vi "dfd_FIR Windowed (Uniform) Filter Coefficients.vi"(6 "sampling freq: fs":dbl=1.0 format="%0.2f", 7 "filter type":T1(ring), 8 "error in (no error)":errorcluster, 9 "low cutoff freq: fl":dbl=0.125 format="%0.2f", 10 "high cutoff freq: fh":dbl=0.45 format="%0.2f", 11 "order":i32=25) -> (0 "error out":errorcluster, 3 "FIR Coefficients":dbl[](array[numeric]) format="%#_2f")   [LabVIEW 2017, in "NI_DigFilter_Design.lvlib"]
doc: "Generates the set of coefficients to implement an FIR filter."
uses:
  <vilib>/addons/Digital Filter Design/NI_DigFilter_Design.lvlib
  <vilib>/Analysis/1siggen.llb/Ramp Pattern by Samples.vi
  <vilib>/Analysis/NI_AALBase.lvlib
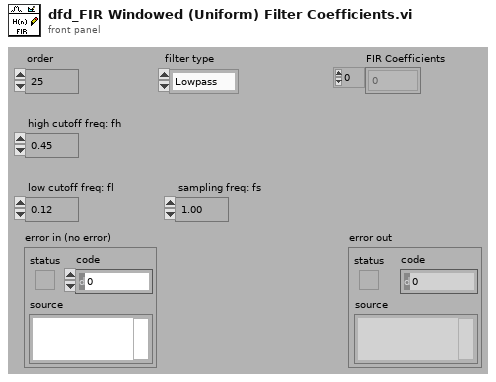
[diagram p1: front panel]
types:
  T1 = enum16{"Lowpass", "Highpass", "Bandpass", "Bandstop"}
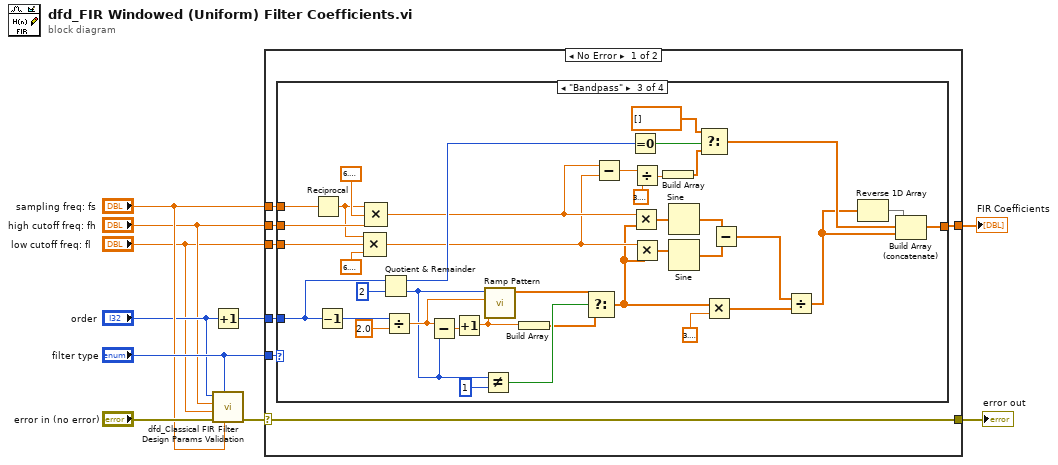
[diagram p0: block diagram]
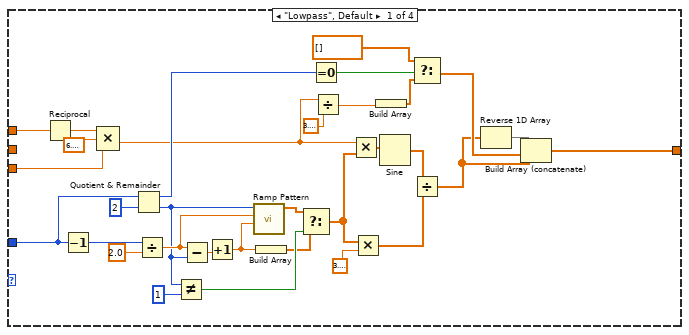
[diagram p2: hidden frame]
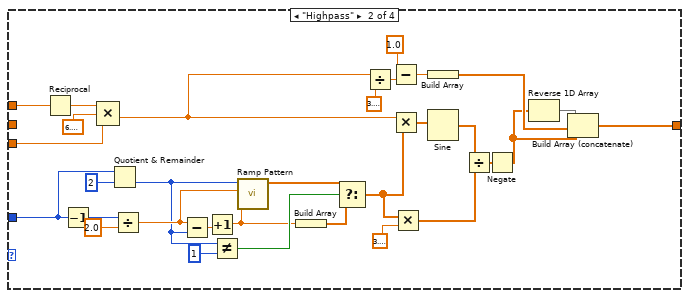
[diagram p3: hidden frame]
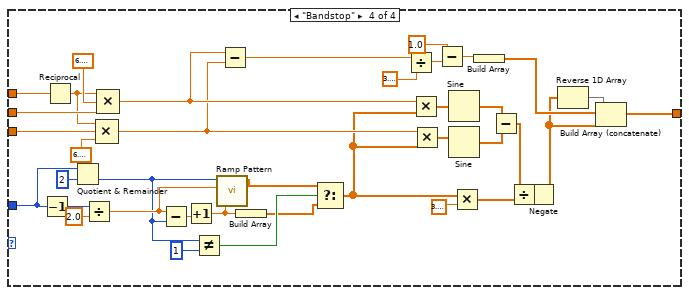
[diagram p4: hidden frame]
diagram:
  n1 = Increment(x="order") -> (x+1=w1:i32)
  n2 = call <vilib>:"dfd_Classical FIR Filter Design Params Validation.vi"("fs [Hz]"="sampling freq: fs", "filter type"="filter type", "error in (no error)"="error in (no error)", "low cutoff freq: fl"="low cutoff freq: fl", "high cutoff freq: fh"="high cutoff freq: fh", "order"="order") -> ("error out"=w3:errorcluster)  [unwired: 5 out]
  n3 = case shown="No Error" w3 {
    selector: w3 -> [w11 w158]
    tunnel: [w17 _] -> w10
    tunnel: "filter type" -> [w16 _]
    tunnel: "sampling freq: fs" -> [w15 _]
    tunnel: w1 -> [w14 _]
    tunnel: "high cutoff freq: fh" -> [w13 _]
    tunnel: "low cutoff freq: fl" -> [w12 _]
    tunnel: [w11 w158] -> w2
    frame No Error {
      n4 = case shown="\"Bandpass\"" w16 {
        tunnel: w15 -> [w49 w80 w117 w155]
        tunnel: w13 -> [_ _ w118 w156]
        tunnel: w14 -> [w45 w76 w82 w145]
        tunnel: [w29 w65 w92 w134] -> w17
        tunnel: w12 -> [w25 w57 w114 w152]
        frame "Lowpass", Default {
          n5 = Reciprocal(x=w49) -> (1/x=w48:dbl)
          n6 = Decrement(x=w45) -> (x-1=w27:i32)
          n7 = Compound Arithmetic op=MULTIPLY(w48, 6.283185307179586, w25) -> (w33:dbl)
          n8 = Quotient & Remainder(x=w45, y=2) -> (x-y*floor(x/y)=w37:i32, floor(x/y)=w24:i32)
          n9 = Divide(x=w27, y=2.0) -> (x/y=w43:dbl)
          n10 = Not Equal?(x=w24, y=1) -> (x != y?=w22:bool)
          n11 = Subtract(x=w43, y=w24) -> (x-y=w42:dbl)
          n12 = Increment(x=w42) -> (x+1=w19:dbl)
          n13 = call-poly <vilib>:"Ramp Pattern.vi"("start"=w19, "end"=w43, "samples"=w24) -> ("Ramp Pattern"=w21:dbl[])  [unwired: 7 in, 1 out]
          n14 = Build Array(w19) -> (w18:dbl[])
          n15 = Select(t=w21, s=w22, f=w18) -> (s? t:f=w20:dbl[])
          n16 = Equal To 0?(x=w37) -> (x = 0?=w36:bool)
          n17 = Divide(x=w33, y=3.141592653589793) -> (x/y=w32:dbl)
          n18 = Multiply(x=w33, y=w20) -> (x*y=w40:dbl[])
          n19 = Multiply(x=w20, y=3.141592653589793) -> (x*y=w38:dbl[])
          n20 = Build Array(w32) -> (w31:dbl[])
          n21 = Sine(x=w40) -> (sin(x)=w39:dbl[])
          n22 = Select(t=dbl[] [], s=w36, f=w31) -> (s? t:f=w30:dbl[])
          n23 = Divide(x=w39, y=w38) -> (x/y=w26:dbl[])
          n24 = Reverse 1D Array(array=w26) -> (reversed array=w28:dbl[])
          n25 = Build Array (concatenate)(w28, w30, w26) -> (w29:dbl[])
        }
        frame "Highpass" {
          n26 = Reciprocal(x=w80) -> (1/x=w79:dbl)
          n27 = Decrement(x=w76) -> (x-1=w62:i32)
          n28 = Compound Arithmetic op=MULTIPLY(w79, 6.283185307179586, w57) -> (w67:dbl)
          n29 = Quotient & Remainder(x=w76, y=2) -> (floor(x/y)=w55:i32)  [unwired: 1 out]
          n30 = Divide(x=w62, y=2.0) -> (x/y=w74:dbl)
          n31 = Subtract(x=w74, y=w55) -> (x-y=w73:dbl)
          n32 = Increment(x=w73) -> (x+1=w51:dbl)
          n33 = Not Equal?(x=w55, y=1) -> (x != y?=w52:bool)
          n34 = call-poly <vilib>:"Ramp Pattern.vi"("start"=w51, "end"=w74, "samples"=w55) -> ("Ramp Pattern"=w53:dbl[])  [unwired: 7 in, 1 out]
          n35 = Build Array(w51) -> (w50:dbl[])
          n36 = Select(t=w53, s=w52, f=w50) -> (s? t:f=w54:dbl[])
          n37 = Divide(x=w67, y=3.141592653589793) -> (x/y=w66:dbl)
          n38 = Subtract(x=1.0 ("y"), y=w66) -> (x-y=w61:dbl)
          n39 = Multiply(x=w67, y=w54) -> (x*y=w71:dbl[])
          n40 = Multiply(x=w54, y=3.141592653589793) -> (x*y=w69:dbl[])
          n41 = Build Array(w61) -> (w59:dbl[])
          n42 = Sine(x=w71) -> (sin(x)=w70:dbl[])
          n43 = Divide(x=w70, y=w69) -> (x/y=w64:dbl[])
          n44 = Negate(x=w64) -> (-x=w58:dbl[])
          n45 = Reverse 1D Array(array=w58) -> (reversed array=w63:dbl[])
          n46 = Build Array (concatenate)(w63, w59, w58) -> (w65:dbl[])
        }
        frame "Bandpass" {
          n47 = Reciprocal(x=w117) -> (1/x=w116:dbl)
          n48 = Decrement(x=w82) -> (x-1=w81:i32)
          n49 = Compound Arithmetic op=MULTIPLY(w116, w114, 6.283185307179586) -> (w90:dbl)
          n50 = Compound Arithmetic op=MULTIPLY(w116, 6.283185307179586, w118) -> (w91:dbl)
          n51 = Quotient & Remainder(x=w82, y=2) -> (x-y*floor(x/y)=w97:i32, floor(x/y)=w88:i32)
          n52 = Divide(x=w81, y=2.0) -> (x/y=w111:dbl)
          n53 = Subtract(x=w111, y=w88) -> (x-y=w112:dbl)
          n54 = Increment(x=w112) -> (x+1=w84:dbl)
          n55 = Not Equal?(x=w88, y=1) -> (x != y?=w85:bool)
          n56 = call-poly <vilib>:"Ramp Pattern.vi"("start"=w84, "end"=w111, "samples"=w88) -> ("Ramp Pattern"=w86:dbl[])  [unwired: 7 in, 1 out]
          n57 = Build Array(w84) -> (w83:dbl[])
          n58 = Select(t=w86, s=w85, f=w83) -> (s? t:f=w87:dbl[])
          n59 = Subtract(x=w91, y=w90) -> (x-y=w96:dbl)
          n60 = Equal To 0?(x=w97) -> (x = 0?=w98:bool)
          n61 = Multiply(x=w91, y=w87) -> (x*y=w108:dbl[])
          n62 = Divide(x=w96, y=3.141592653589793) -> (x/y=w101:dbl)
          n63 = Multiply(x=w90, y=w87) -> (x*y=w107:dbl[])
          n64 = Build Array(w101) -> (w102:dbl[])
          n65 = Sine(x=w108) -> (sin(x)=w106:dbl[])
          n66 = Sine(x=w107) -> (sin(x)=w105:dbl[])
          n67 = Select(t=dbl[] [], s=w98, f=w102) -> (s? t:f=w94:dbl[])
          n68 = Multiply(x=w87, y=3.141592653589793) -> (x*y=w103:dbl[])
          n69 = Subtract(x=w106, y=w105) -> (x-y=w104:dbl[])
          n70 = Divide(x=w104, y=w103) -> (x/y=w93:dbl[])
          n71 = Reverse 1D Array(array=w93) -> (reversed array=w95:dbl[])
          n72 = Build Array (concatenate)(w95, w94, w93) -> (w92:dbl[])
        }
        frame "Bandstop" {
          n73 = Decrement(x=w145) -> (x-1=w151:i32)
          n74 = Reciprocal(x=w155) -> (1/x=w154:dbl)
          n75 = Quotient & Remainder(x=w145, y=2) -> (floor(x/y)=w127:i32)  [unwired: 1 out]
          n76 = Divide(x=w151, y=2.0) -> (x/y=w148:dbl)
          n77 = Compound Arithmetic op=MULTIPLY(w154, w152, 6.283185307179586) -> (w132:dbl)
          n78 = Compound Arithmetic op=MULTIPLY(w154, 6.283185307179586, w156) -> (w133:dbl)
          n79 = Subtract(x=w148, y=w127) -> (x-y=w149:dbl)
          n80 = Increment(x=w149) -> (x+1=w123:dbl)
          n81 = Not Equal?(x=w127, y=1) -> (x != y?=w124:bool)
          n82 = call-poly <vilib>:"Ramp Pattern.vi"("start"=w123, "end"=w148, "samples"=w127) -> ("Ramp Pattern"=w126:dbl[])  [unwired: 7 in, 1 out]
          n83 = Subtract(x=w133, y=w132) -> (x-y=w137:dbl)
          n84 = Build Array(w123) -> (w122:dbl[])
          n85 = Select(t=w126, s=w124, f=w122) -> (s? t:f=w125:dbl[])
          n86 = Divide(x=w137, y=3.141592653589793) -> (x/y=w139:dbl)
          n87 = Multiply(x=w133, y=w125) -> (x*y=w144:dbl[])
          n88 = Multiply(x=w132, y=w125) -> (x*y=w143:dbl[])
          n89 = Subtract(x=1.0, y=w139) -> (x-y=w130:dbl)
          n90 = Sine(x=w144) -> (sin(x)=w142:dbl[])
          n91 = Sine(x=w143) -> (sin(x)=w141:dbl[])
          n92 = Multiply(x=w125, y=3.141592653589793) -> (x*y=w140:dbl[])
          n93 = Build Array(w130) -> (w131:dbl[])
          n94 = Subtract(x=w142, y=w141) -> (x-y=w121:dbl[])
          n95 = Divide(x=w121, y=w140) -> (x/y=w135:dbl[])
          n96 = Negate(x=w135) -> (-x=w120:dbl[])
          n97 = Reverse 1D Array(array=w120) -> (reversed array=w136:dbl[])
          n98 = Build Array (concatenate)(w136, w131, w120) -> (w134:dbl[])
        }
      }
    }
    frame Error {
    }
  }
  "FIR Coefficients" <- w10
  "error out" <- w2
